vi "8-5 화상키보드 실행.vi"() -> ()   [LabVIEW 2014]
panel:
  in  "정지":bool
  in  "screen Keyboard":bool
  in  "문자열 입력":string
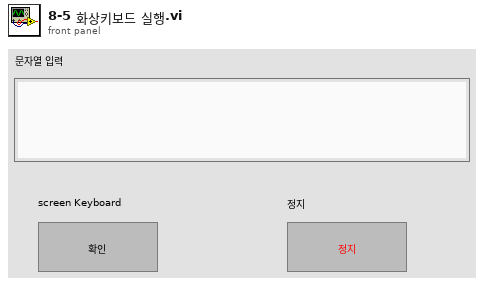
[diagram p1: front panel]
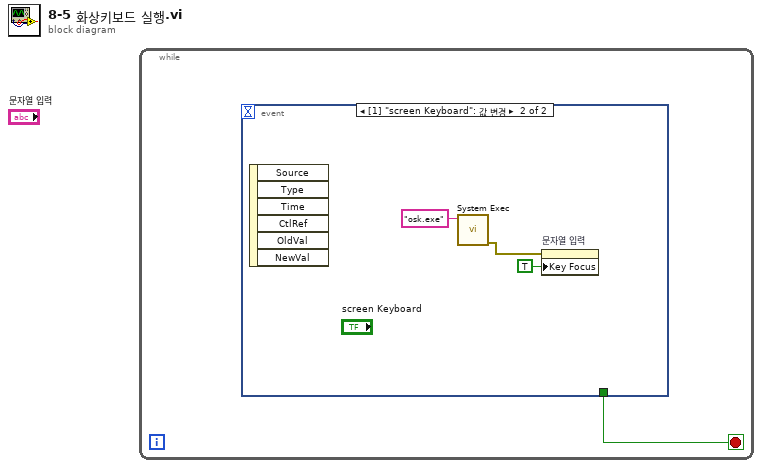
[diagram p0: block diagram]
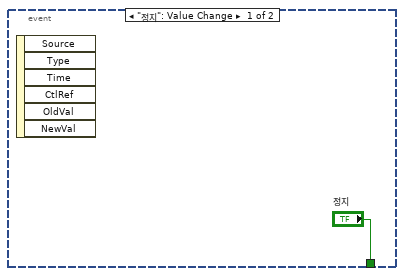
[diagram p2: hidden frame]
diagram:
  n1 = while {
    stop <- w1 stop-if-true
    n2 = event shown="[1] \"screen Keyboard\": 값 변경" {
      selector: _ -> [_ _]
      dyn-events: _ -> [_ _]
      timeout: _ -> [_ _]
      tunnel: ["정지" _] -> w1
      event "정지": Value Change {
        n3 = event-data() -> ()  [unwired: 1 in, 6 out]
      }
      event "screen Keyboard": Value Change {
        n4 = event-data() -> ()  [unwired: 1 in, 6 out]
        n5 = call <vilib>:"System Exec.vi"("command line"="osk.exe") -> ("error out"=w3:errorcluster)  [unwired: 7 in, 3 out]
        n6 = property on="문자열 입력" class="Str"(error in=w3, "Key Focus"=TRUE ("키 포커스")) -> ()  [unwired: 1 in, 2 out]
      }
    }
  }
